vi "Get Channel Specification Page Settings.vi"(8 "error in":errorcluster, 11 "parameter ref":T3 format="%.0x") -> (0 "error out":errorcluster, 1 "Channel":T1, 2 "Channel Settings":string[](array[string]), 3 "parameter ref out":T3 format="%.0x")   [LabVIEW 2024, in "AIM ARINC 429 Scripting.lvlib"]
uses:
  AIM ARINC 429 Scripting.lvlib
  <vilib>/NI VeriStand/Custom Device API/Custom Device Item Ref.ctl
  <vilib>/NI VeriStand/Custom Device API/Custom Device Channel.ctl
  <vilib>/NI VeriStand/Custom Device API/Custom Device Channel Type.ctl
  <vilib>/NI VeriStand/Custom Device API/Custom Device API.lvlib
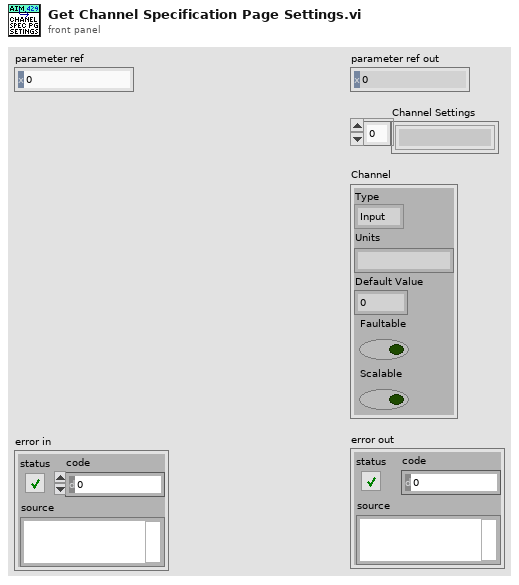
[diagram p1: front panel]
types:
  T1 = typedef "Custom Device API.lvlib/Custom Device Channel.ctl" = cluster{"Type":T2, "Units":string, "Default Value":dbl, "Faultable":bool, "Scalable":bool}
  T2 = typedef "Custom Device API.lvlib/Custom Device Channel Type.ctl" = enum16{"Input", "Output"}
  T3 = typedef "Custom Device API.lvlib/Custom Device Item Ref.ctl" = u64
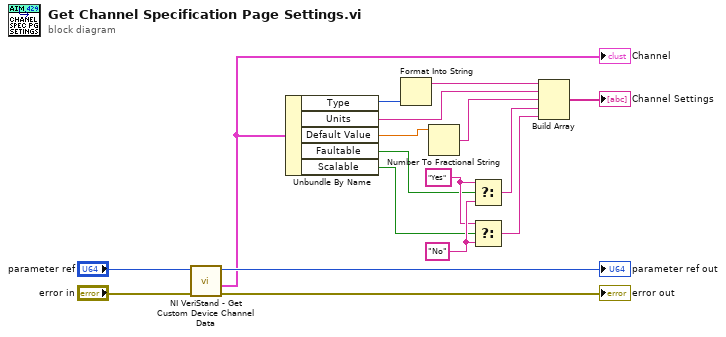
[diagram p0: block diagram]
diagram:
  w11 = "No"
  w10 = "Yes"
  n1 = call <vilib>:"NI VeriStand - Get Custom Device Channel Data.vi"("error in (no error)"="error in", "Channel Ref in"="parameter ref") -> ("error out"=→"error out":errorcluster, "Channel"=w2:T1, "Channel Ref out"=→"parameter ref out":T3)  [unwired: 4 in, 3 out]
  "Channel" <- w2
  n2 = Unbundle By Name(w2) -> ("Type"=w12:T2, "Units"=w5:string, "Default Value"=w13:dbl, "Faultable"=w7:bool, "Scalable"=w1:bool)
  n3 = Format Into String(w12) -> (resulting string=w4:string)  [unwired: 3 in, 1 out]
  n4 = Number To Fractional String(number=w13) -> (F-format string=w6:string)  [unwired: 3 in]
  n5 = Select(t=w10, s=w7, f=w11) -> (s? t:f=w8:string)
  n6 = Select(t=w10, s=w1, f=w11) -> (s? t:f=w9:string)
  n7 = Build Array(w4, w5, w6, w8, w9) -> (→"Channel Settings":string[])
